vi "Scrape Screenpops.vi"(8 "error in":errorcluster, 11 "SR number list in":i32[](array[numeric])) -> (0 "error out":errorcluster, 3 "sr clusters out":T2[](array[typedef]) {"Creation Date" format="%<%x>T"; "Last Updated" format="%<%x>T"})   [LabVIEW 2018]
uses:
  Type Defs/SR Cluster.ctl
  Type Defs/SR Status.ctl
  Type Defs/SR Note Cluster.ctl
  <vilib>/httpClient/LabVIEWHTTPClient.lvlib
panel:
  out "body":string
  out "sr notes array out":T1[][](array[typedef]) {"Note Date" format="%<%x >T"}
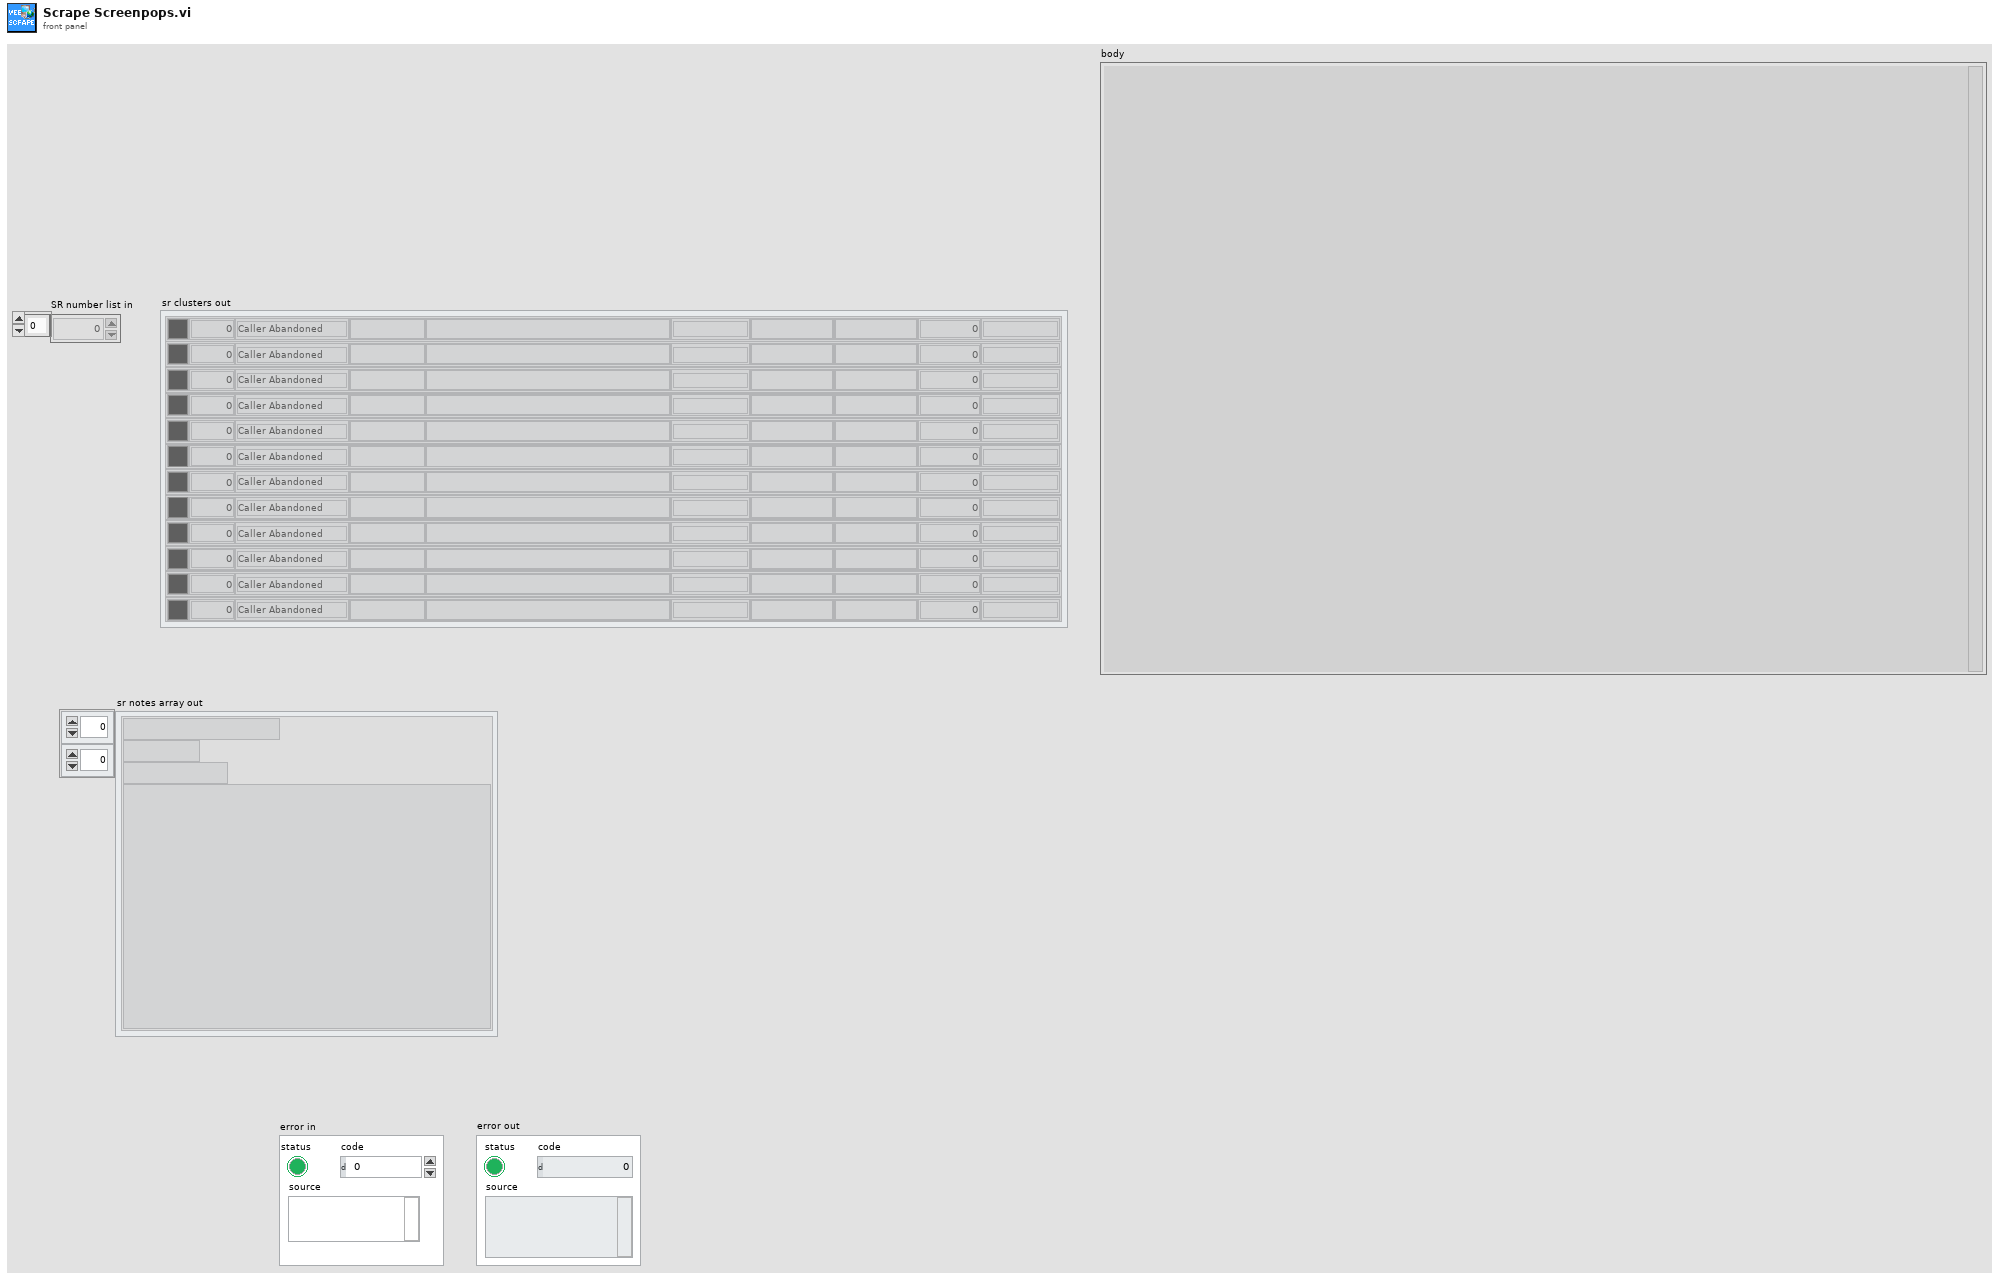
[diagram p1: front panel]
types:
  T1 = typedef "SR Note Cluster.ctl" = cluster{"Note Type":string, "Note Date":timestamp, "AE":string, "Note Text":string}
  T2 = typedef "SR Cluster.ctl" = cluster{"Color":u32, "SR Number":i32, "SR Status":T3, "Name":string, "Summary":string, "Last Updated":timestamp, "SR Type":string, "Service Level":string, "Days Open":dbl, "Creation Date":timestamp}
  T3 = typedef "SR Status.ctl" = enum16{"Caller Abandoned", "Created in Error", "Expired", "Forum Resolved AE", "Forum Resolved Customer", "IN WORK", "IN WORK Collab with AES", "IN WORK Collab with PSE", "IN WORK Collab with SE", "IN WORK Customer Added Note", "IN WORK Escalation", "IN WORK Wait on Customer", "Open", "Potentially Resolved", "Presumed Resolved", "RMA Approved for Return", "Resolved", "Passed Off"}
  T4 = typedef "LabVIEWHTTPClient.lvlib/ClientHandle.ctl" = refnum<k1>
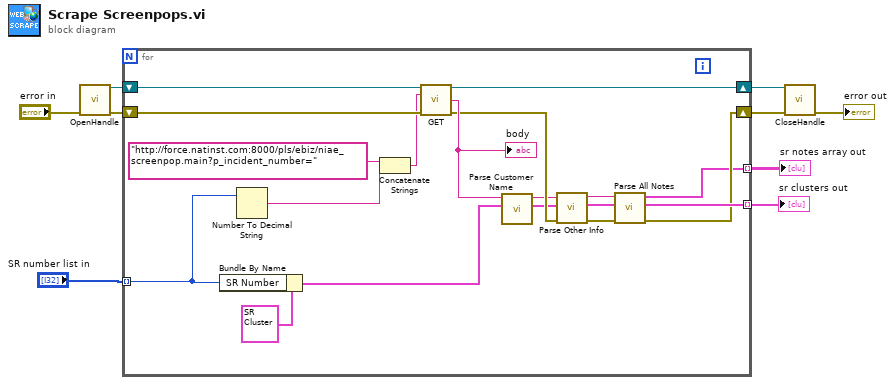
[diagram p0: block diagram]
diagram:
  n1 = call <vilib>:"OpenHandle.vi"("error in (no error)"="error in") -> ("client handle out"=w9:T4, "error out"=w8:errorcluster)  [unwired: 13 in]
  n2 = for {
    tunnel: "SR number list in" -> [w21] mode=indexing
    tunnel: [w23] -> w5 mode=indexing
    tunnel: [w19] -> w1 mode=indexing
    shift-right: [w10] -> w7
    shift-left: w9 -> [w28]
    shift-right: [w20] -> w6
    shift-left: w8 -> [w27]
    n3 = Bundle By Name(cluster=T2 {"Color"=0, "SR Number"=0, "SR Status"=enum."Caller Abandoned", "Name"="", "Summary"="", "Last Updated"=timestamp(0 s since 1904-01-01), "SR Type"="", "Service Level"="", "Days Open"=0.0, "Creation Date"=timestamp(0 s since 1904-01-01)} ("SR Cluster"), "SR Number"=w21) -> (w17:T2)
    n4 = Number To Decimal String(number=w21) -> (decimal integer string=w26:string)  [unwired: 1 in]
    n5 = Concatenate Strings("http://force.natinst.com:8000/pls/ebiz/niae_screenpop.main?p_incident_number=" ("string"), w26) -> (w25:string)
    n6 = call <vilib>:"GET.vi"("client handle"=w28, "url"=w25, "error in (no error)"=w27) -> ("client handle out"=w10:T4, "body"=w18:string, "error out"=w16:errorcluster)  [unwired: 9 in, 1 out]
    "body" <- w18
    n7 = call "Parse Customer Name.vi"("SR Cluster in"=w17, "HTML text in"=w18) -> ("SR Cluster out"=w15:T2, "remaining string out"=w14:string)  [unwired: 8 in]
    n8 = call "Parse Other Info.vi"("error in (no error)"=w16, "SR Cluster in"=w15, "remaining string in"=w14) -> ("error out"=w11:errorcluster, "SR Cluster out 2"=w12:T2, "result string"=w13:string)  [unwired: 6 in]
    n9 = call "Parse All Notes.vi"("error in (no error)"=w11, "SR Cluster in"=w12, "result string"=w13) -> ("error out"=w20:errorcluster, "SR Cluster out"=w23:T2, "Array"=w19:T1[])  [unwired: 6 in]
  }
  "sr clusters out" <- w5
  "sr notes array out" <- w1
  n10 = call <vilib>:"CloseHandle.vi"("client handle"=w7, "error in (no error)"=w6) -> ("error out"=→"error out":errorcluster)  [unwired: 13 in]
